vi "Test Resampling.vi"() -> ()   [LabVIEW 2019, in "Instrument.Lockin.lvlib" / "Instrument.DAQ.lvclass"]
uses:
  Instrument.DAQ.lvclass
  DAQmx/DAQmx.lvclass
  DSP/DSP.lvclass
  <vilib>/measure/NI_MABase.lvlib
  <vilib>/Waveform/WDTOps.llb/WDT Number of Waveform Samples DBL.vi
  <vilib>/ptbypt/NI_PtbyPt.lvlib
panel:
  out "Array":i32[](array[numeric])
  out "Numeric":i32
  in  "stop":bool
  out "<time (s)>":dbl format="%#_6p"
  in  "sampling info":cluster{"Fs":dbl, "#s":dbl}={"Fs"=1000.0, "#s"=1000.0}
  out "Waveform Graph":waveform(dbl)[](graph)
  in  "frequency":dbl[](array[numeric]) format="%0.2p"
  in  "output fs[Hz]":dbl=6500.0 format="%#_13g"
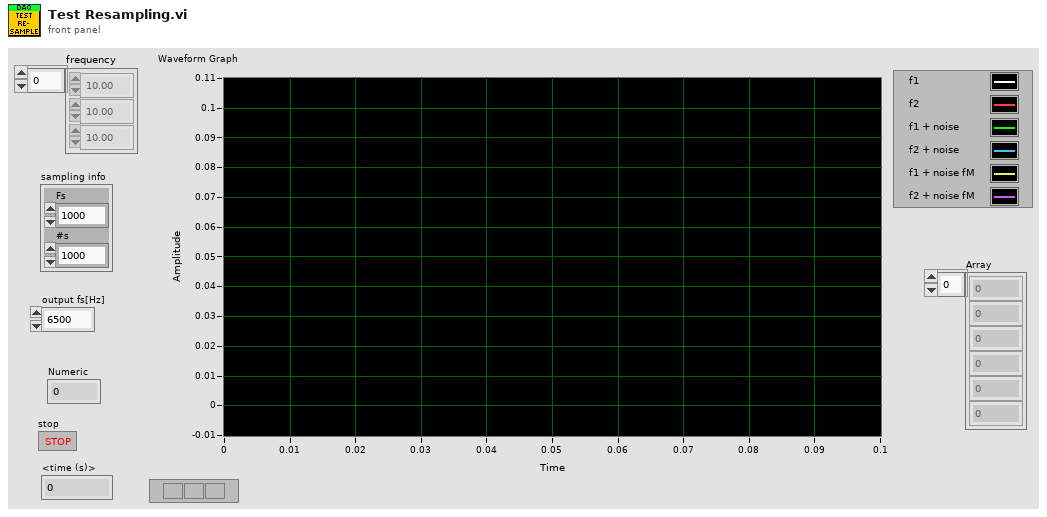
[diagram p1: front panel]
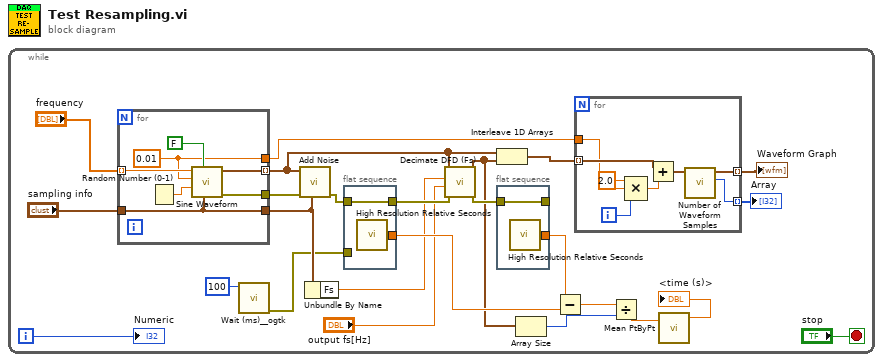
[diagram p0: block diagram]
diagram:
  n1 = while {
    i -> [w16]
    stop <- "stop" stop-if-true
    n2 = for {
      tunnel: [w44] -> w12 mode=indexing
      tunnel: "sampling info" -> [w43]
      tunnel: [w43] -> w11
      tunnel: [w42] -> w25
      tunnel: "frequency" -> [w41] mode=indexing
      tunnel: [w38] -> w13
      w38 = 0.01 ("amplitude")
      n3 = Random Number (0-1)() -> (number: 0 to 1=w39:dbl)
      n4 = call <vilib>:"Sine Waveform.vi"("sampling info"=w43, "reset signal"=FALSE, "phase"=w39, "amplitude"=w38, "frequency"=w41) -> ("error out"=w42:errorcluster, "signal out"=w44:waveform(dbl))  [unwired: 5 in]
    }
    n5 = call <userlib>:"Wait (ms)__ogtk.vi"("milliseconds to wait"=u32 100) -> ("error out"=w9:errorcluster)  [unwired: 9 in, 1 out]
    n6 = call "Add Noise.vi"("Sampling"=w11, "error in (no error)"=w25, "AI []"=w12) -> ("error out"=w22:errorcluster)  [unwired: 7 in, 1 out]
    n7 = Unbundle By Name(w11) -> ("Fs"=w8:dbl)
    n8 = flat-sequence {
      tunnel: w22 -> [w29]
      tunnel: [w29] -> w21
      tunnel: [w28] -> w18
      tunnel: w9 -> [_]
      frame #0 {
        n9 = call <vilib>:"High Resolution Relative Seconds.vi"() -> ("relative seconds"=w28:dbl)
      }
    }
    n10 = call "Decimate DFD (Fs).vi"("error in (no error)"=w21, "output fs (Hz)"="output fs[Hz]", "Fs"=w8, "Waveforms in"=w12) -> ("error out"=w20:errorcluster, "waveforms out"=w6:waveform(dbl)[])  [unwired: 6 in]
    n11 = Interleave 1D Arrays(w12, w6) -> (w24:waveform(dbl)[])
    n12 = flat-sequence {
      tunnel: w20 -> [w27]
      tunnel: [w27] -> _
      tunnel: [w26] -> w19
      frame #0 {
        n13 = call <vilib>:"High Resolution Relative Seconds.vi"() -> ("relative seconds"=w26:dbl)
      }
    }
    n14 = Array Size(array=w6) -> (size(s)=w5:i32)
    n15 = Subtract(x=w19, y=w18) -> (x-y=w4:dbl)
    n16 = for {
      tunnel: w24 -> [w35] mode=indexing
      tunnel: [w30] -> w23 mode=indexing
      tunnel: w13 -> [w34]
      tunnel: [w32] -> w7 mode=indexing
      i -> [w37]
      n17 = Compound Arithmetic op=MULTIPLY(2.0 ("value"), w34, w37) -> (w36:dbl)
      n18 = Add(x=w35, y=w36) -> (x+y=w31:waveform(dbl))
      n19 = call-poly <vilib>:"Number of Waveform Samples.vi"("waveform in"=w31) -> ("number of samples"=w32:i32, "waveform out"=w30:waveform(dbl))  [unwired: 8 in, 1 out]
    }
    "Waveform Graph" <- w23
    "Array" <- w7
    n20 = Divide(x=w4, y=w5) -> (x/y=w3:dbl)
    n21 = call <vilib>:"Mean PtByPt.vi"("x"=w3) -> ("mean"=→"<time (s)>":dbl)  [unwired: 3 in, 1 out]
    "Numeric" <- w16
  }
